vi "CLSUIP_GetFPTermFromTerminal.vi"(2 "error in (no error)":errorcluster, 3 "Term Refnum":refnum<vi>) -> (0 "error out":errorcluster, 1 "CtrlTerm Refnum":refnum<vi>)   [LabVIEW 2021, in "MemberVICreation.lvlib" / "VIRetooler.lvclass"]
uses:
  <resource>/Framework/Providers/LVClassLibrary/NewAccessors/VIRetooler/VIRetooler.lvclass
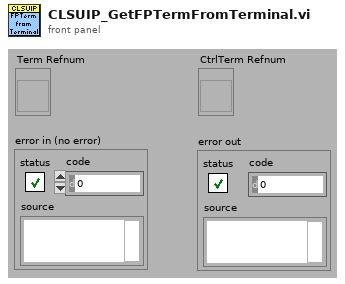
[diagram p1: front panel]
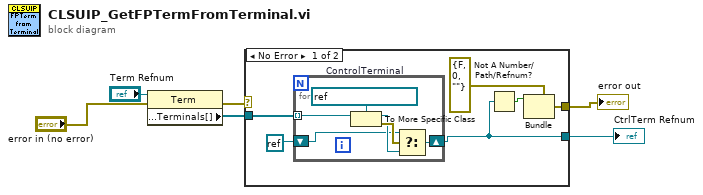
[diagram p0: block diagram]
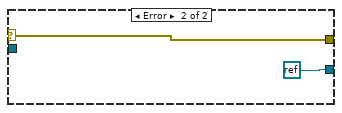
[diagram p2: hidden frame]
diagram:
  n1 = property class="Term"(reference="Term Refnum", error in="error in (no error)") -> (error out=w2:errorcluster, "Connected Wire.Terminals[]"=w5:refnum<vi>[])  [unwired: 1 out]
  n2 = case shown="No Error" w2 {
    selector: w2 -> [_ w20]
    tunnel: [w10 refnum<k0> refnum] -> w6
    tunnel: w5 -> [w11 _]
    tunnel: [w7 w20] -> w1
    frame No Error {
      n3 = for {
        tunnel: w11 -> [w17] mode=indexing
        shift-right: [w13] -> w10
        shift-left: refnum<k0> refnum -> [w14]
        w18 = refnum<vi> refnum  # ControlTerminal
        n4 = To More Specific Class(target class=w18, reference=w17) -> (specific class reference=w15:refnum<vi>, error out=w16:errorcluster)  [unwired: 1 in]
        n5 = Select(t=w14, s=w16, f=w15) -> (s? t:f=w13:refnum<vi>)
      }
      n6 = Not A Number/Path/Refnum?(number/path/refnum=w10) -> (NaN/Path/Refnum?=w8:bool)
      n7 = Bundle(cluster=errorcluster {"status"=FALSE, "code"=0, "source"=""} ("error IO"), "status"=w8) -> (w7:errorcluster)  [unwired: 2 out]
    }
    frame Error {
    }
  }
  "CtrlTerm Refnum" <- w6
  "error out" <- w1
